vi "Motor_check.vi"() -> (0 "error out":errorcluster, 1 "steps per degree out":dbl=1.67, 2 "reply":string, 3 "VISA Refnum out":refnum<visa-resource-name>)   [LabVIEW 2022 SP3]
uses:
  <vilib>/Instr/_visa.llb/VISA Configure Serial Port (Instr).vi
panel:
  out "steps":i32
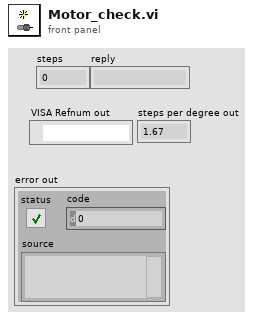
[diagram p1: front panel]
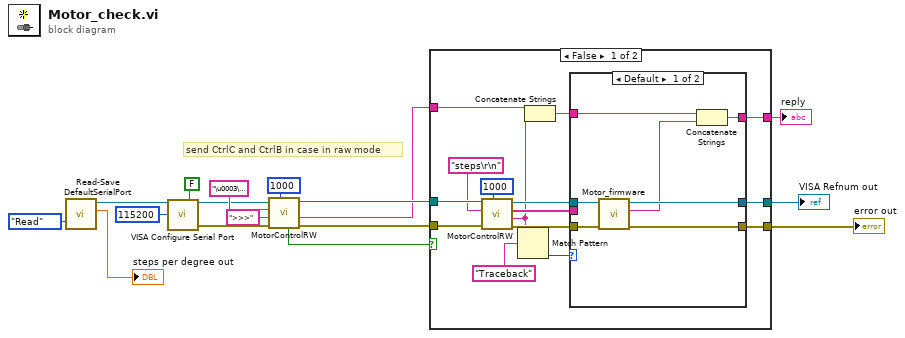
[diagram p0: block diagram]
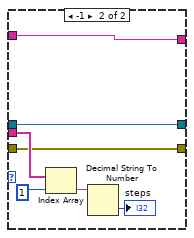
[diagram p2: hidden frame]
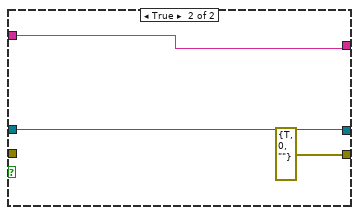
[diagram p3: hidden frame]
diagram:
  # "send CtrlC and CtrlB in case in raw mode"
  n1 = call "Read-Save DefaultSerialPort.vi"("Task"=enum16{"Save", "Read"}."Read") -> ("steps per degree out"=→"steps per degree out":dbl, "VISA out"=w16:refnum<visa-resource-name>)  [unwired: 8 in, 1 out]
  n2 = call-poly "VISA Configure Serial Port"("VISA resource name"=w16, "Enable Termination\nChar (T)"=FALSE ("Enable Termination\nChar (T)"), "baud rate (9600)"=u32 115200) -> ("VISA resource name out"=w10:refnum<visa-resource-name>, "error out"=w9:errorcluster)  [unwired: 11 in]
  n3 = call "MotorControlRW.vi"("timeout (msec)"=u32 1000, "error in (no error)"=w9, "end"=">>>", "payload"="\u0003\u0002" ("element"), "VISA in"=w10) -> ("error out"=w6:errorcluster, "reply"=w3:string, "VISA Out"=w7:refnum<visa-resource-name>, "Timed out"=w8:bool)  [unwired: 2 in, 1 out]
  n4 = case shown="False" w8 {
    tunnel: w7 -> [w31 w48]
    tunnel: w6 -> [w30 _]
    tunnel: [w23 errorcluster {"status"=TRUE, "code"=0, "source"=""} ("error out")] -> w5
    tunnel: [w22 w48] -> w4
    tunnel: w3 -> [w21 w46]
    tunnel: [w18 w46] -> w2
    frame False {
      n5 = call "MotorControlRW.vi"("timeout (msec)"=u32 1000, "error in (no error)"=w30, "payload"="steps\r\n" ("element"), "VISA in"=w31) -> ("error out"=w24:errorcluster, "reply"=w20:string, "rows"=w28:string[], "VISA Out"=w25:refnum<visa-resource-name>)  [unwired: 3 in, 1 out]
      n6 = Match Pattern(string=w20, regular expression="Traceback" ("element")) -> (offset past match=w26:i32)  [unwired: 1 in, 3 out]
      n7 = Concatenate Strings(w21, w20) -> (w19:string)
      n8 = case shown="Default" w26 {
        tunnel: w28 -> [_ w43]
        tunnel: w25 -> [w36 w41]
        tunnel: w24 -> [w38 w40]
        tunnel: [w37 w40] -> w23
        tunnel: [w36 w41] -> w22
        tunnel: w19 -> [w35 w39]
        tunnel: [w33 w39] -> w18
        frame Default {
          n9 = call "Motor_firmware.vi"("error in (no error)"=w38, "VISA Refnum in"=w36) -> ("error out"=w37:errorcluster, "reply"=w34:string)  [unwired: 8 in]
          n10 = Concatenate Strings(w35, w34) -> (w33:string)
        }
        frame -1 {
          n11 = Index Array(array=w43, index=1) -> (element=w45:string)
          n12 = Decimal String To Number(string=w45) -> (number=→"steps":i32)  [unwired: 2 in, 1 out]
        }
      }
    }
    frame True {
    }
  }
  "error out" <- w5
  "VISA Refnum out" <- w4
  "reply" <- w2
